vi "Insert Important Module VIs.vi"(7 "Application in":refnum<vi>, 8 "Tree Map in":T1, 9 "Root path":string, 10 "DQMH Lib In":refnum<vi>, 11 "map ref in in":map{string, refnum<vi>}(c390)) -> (0 "Tree Map Out":T1, 3 "map ref out":map{string, refnum<vi>}(c390))   [LabVIEW 2019, in "Panther Dashboard.lvlib"]
uses:
  Panther Dashboard.lvlib
  <vilib>/National Instruments/Tree Map/Tree Map Data.ctl
  <vilib>/National Instruments/Tree Map/Tree Map.lvlib
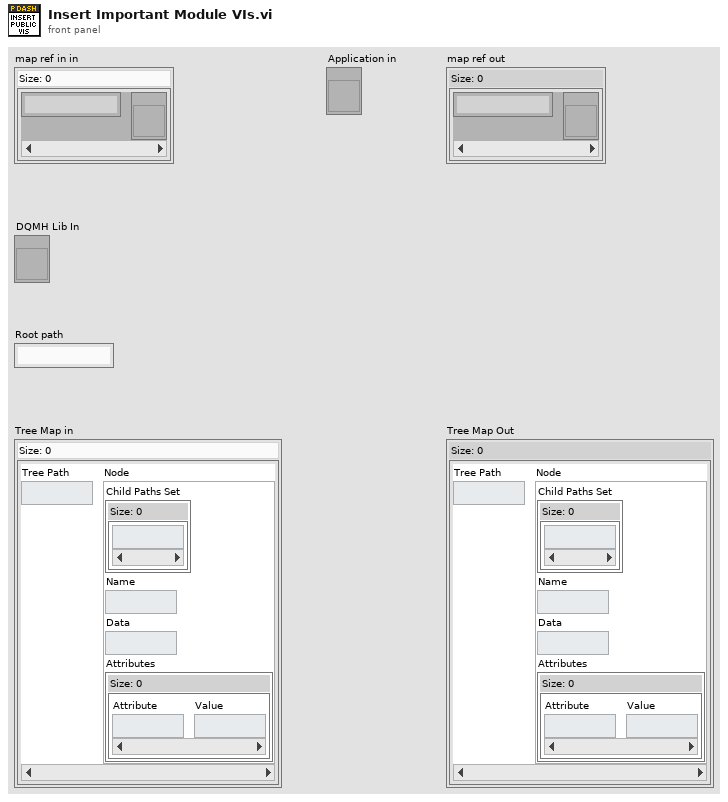
[diagram p1: front panel]
types:
  T1 = typedef "Tree Map.lvlib/Tree Map Data.ctl" = map{string, cluster{"Child Paths Set":set{string}, "Name":string, "Data":string, "Attributes":map{string, string}}}
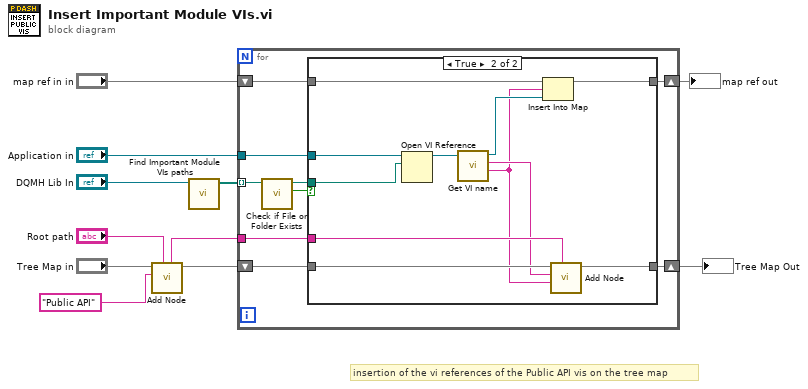
[diagram p0: block diagram]
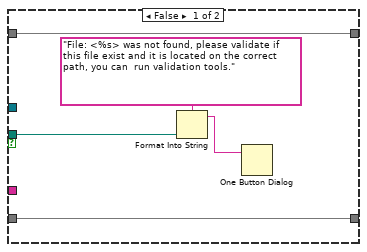
[diagram p2: hidden frame]
diagram:
  # "insertion of the vi references of the Public API vis on the tree map"
  n1 = call <vilib>:"Add Node.vi"("Parent Path"="Root path", "New Node Name"="Public API", "Tree Map In"="Tree Map in") -> ("Tree Map Out"=w3:T1, "New Node Path"=w1:string)  [unwired: 6 in, 1 out]
  n2 = call "Find Important Module VIs paths.vi"("Library in"="DQMH Lib In") -> ("Public API VIs Paths"=w10:path[])  [unwired: 10 in]
  n3 = for {
    tunnel: "Application in" -> [w20]
    tunnel: w10 -> [w14] mode=indexing
    shift-right: [w18] -> w8
    shift-left: "map ref in in" -> [w17]
    shift-right: [w19] -> w9
    shift-left: w3 -> [w16]
    tunnel: w1 -> [w15]
    n4 = call <vilib>:"Check if File or Folder Exists.vi"("path"=w14) -> ("file or folder exists?"=w13:bool, "dup path"=w12:path)  [unwired: 8 in, 1 out]
    n5 = case shown="True" w13 {
      tunnel: w20 -> [_ w36]
      tunnel: [w24 w35] -> w19
      tunnel: [w25 w34] -> w18
      tunnel: w17 -> [w25 w33]
      tunnel: w16 -> [w24 w32]
      tunnel: w15 -> [_ w31]
      tunnel: w12 -> [w23 w26]
      frame False {
        n6 = Format Into String(format string="File: <%s> was not found, please validate if this file exist and it is located on the correct path, you can  run validation tools.", w23) -> (resulting string=w22:string)  [unwired: 2 in, 1 out]
        n7 = One Button Dialog(message=w22) -> ()  [unwired: 1 in, 1 out]
      }
      frame True {
        n8 = Open VI Reference(application reference (local)=w36, vi path=w26) -> (vi reference=w29:refnum<vi>)  [unwired: 4 in, 1 out]
        n9 = call "Get VI name.vi"("VI in"=w29) -> ("Full Vi Name"=w27:string, "Plain Name"=w30:string, "VI out"=w28:refnum<vi>)  [unwired: 8 in]
        n10 = Insert Into Map(map in=w33, key=w27, value=w28) -> (map out=w34:map{string, refnum<vi>})  [unwired: 2 out]
        n11 = call <vilib>:"Add Node.vi"("Parent Path"=w31, "Data"=w27, "New Node Name"=w30, "Tree Map In"=w32) -> ("Tree Map Out"=w35:T1)  [unwired: 5 in, 2 out]
      }
    }
  }
  "Tree Map Out" <- w9
  "map ref out" <- w8
